vi "measureEchoes_anySet.vi"(3 "Read freqs. \nfrom textfile":bool, 5 "Cluster":T1={"span"=600000000.0, "rbw"=1000.0, "enableVBW"=FALSE, "vbw"=0.0, "traceLength"=64001, "window"=0, "verticalUnit"=0, "center freq"=300000000.0} {"verticalUnit" items=["SpectrumVerticalUnit_dBm", "SpectrumVerticalUnit_Watt", "SpectrumVerticalUnit_Volt", "SpectrumVerticalUnit_Amp", "SpectrumVerticalUnit_dBmV"]; "window" items=["SpectrumWindow_Kaiser", "SpectrumWindow_Mil6dB", "SpectrumWindow_BlackmanHarris", "SpectrumWindow_Rectangle", "SpectrumWindow_FlatTop", "SpectrumWindow_Hann"]; "traceLength" items=["801"=801, "2401"=2401, "4001"=4001, "8001"=8001, "10401"=10401, "16001"=16001, "32001"=32001, "64001"=64001]}, 6 "error in":errorcluster, 7 "Echo measurement time":i32=30, 8 "Burn time/OFC measurement time":i32=30, 9 "Folder for all data (Don't forget the last slash!)":string) -> (0 "error out":errorcluster)   [LabVIEW 2016]
uses:
  <vilib>/Utility/file.llb/Read Delimited Spreadsheet (DBL).vi
  <vilib>/Utility/file.llb/Write Delimited Spreadsheet (DBL).vi
panel:
  out "Last saved trace":sgl[](graph)
  in  "stop":bool
  out "RSA error out":errorcluster
  out "Real-time trace":sgl[](graph)
  out "Current set #":i32
  out "Current freq.":dbl
  in  "freqs. file":path
  in  "Shuffle?":bool
  in  "Start freq":dbl=100000.0 format="%0.2e"
  in  "End freq":dbl=20000000.0 format="%0.2e"
  in  "Freq step":i32=100000 format="%.2e"
  in  "Mod shape":enum16{"Triangle", "Sine"}(ring)
  # "RSA settings"
  # "Suppose you want to collect comb data, first ascending, then descending.\n\nIn Matlab, create a 1xM array \ncontaining all modulation freqs (Hz) in the ascending sequence; then create a 1xN array for the descending case. Note that M != N is fine.\n\nfid= fopen(FILENAME, 'w');\nfprintf(fid,'%d\\t', ARRAY1);\nfprintf(fid,'\\r\\n');\nfprintf(fid,'%d\\t',ARRAY2);\n... \n(for more sets, repeat as needed)\nfclose(fid);\n\nNow find the file you just made:"
  # "Modulation settings"
  # "(zero-indexed)"
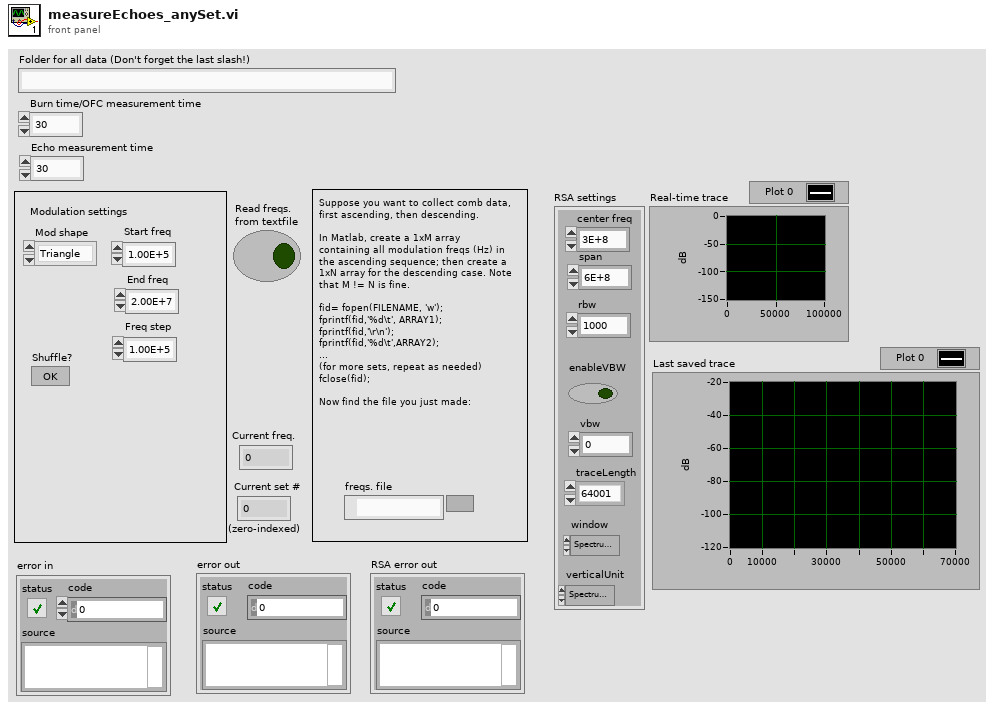
[diagram p1: front panel]
types:
  T1 = cluster{"span":dbl, "rbw":dbl, "enableVBW":bool, "vbw":dbl, "traceLength":u16, "window":u32, "verticalUnit":u32, "center freq":dbl}
  T2 = cluster{"span":dbl, "rbw":dbl, "enableVBW":bool, "vbw":dbl, "traceLength":u16, "window":u32, "verticalUnit":u32}
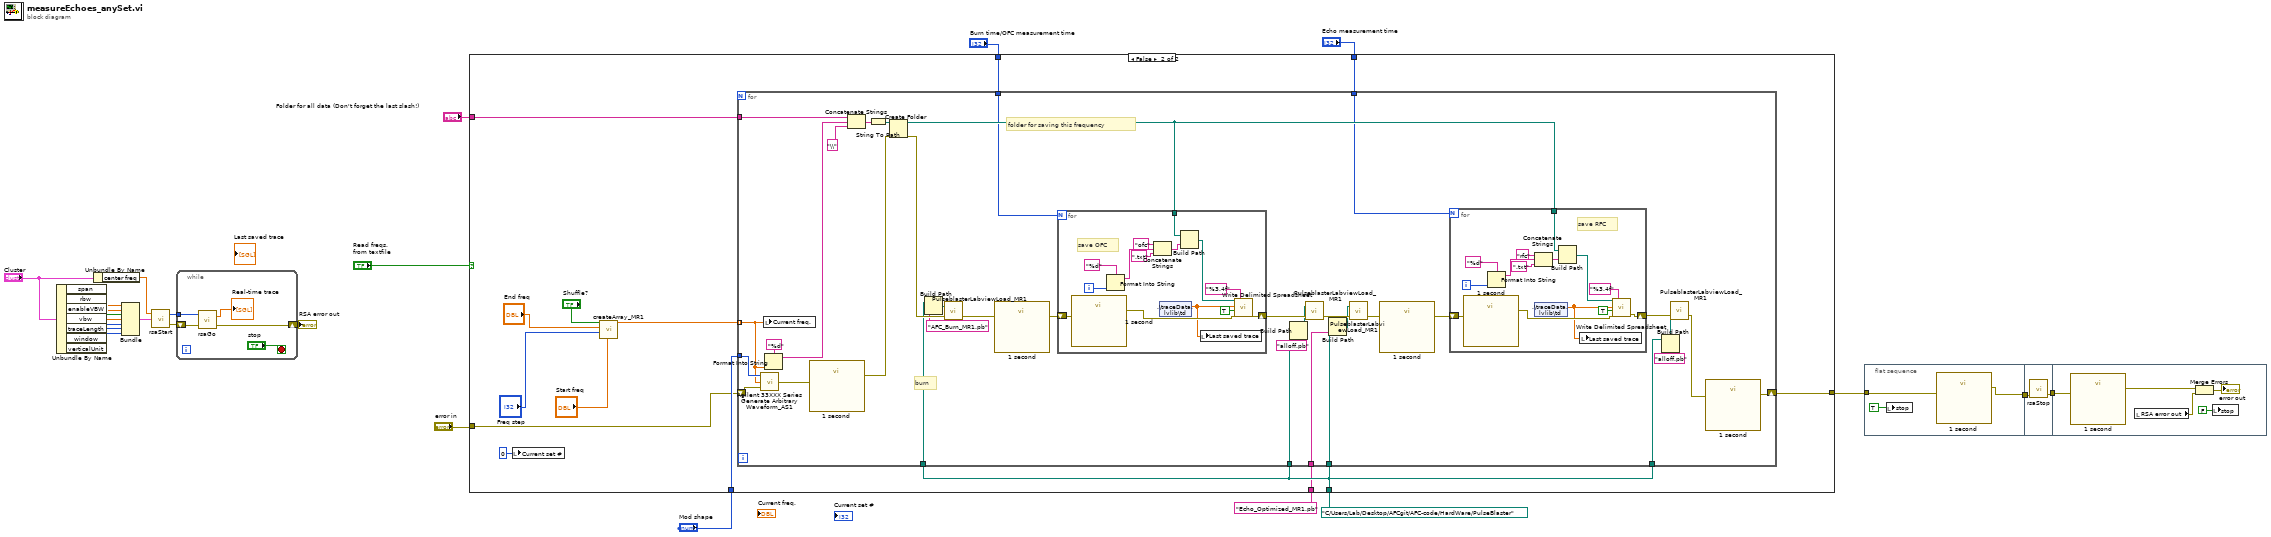
[diagram p0: block diagram]
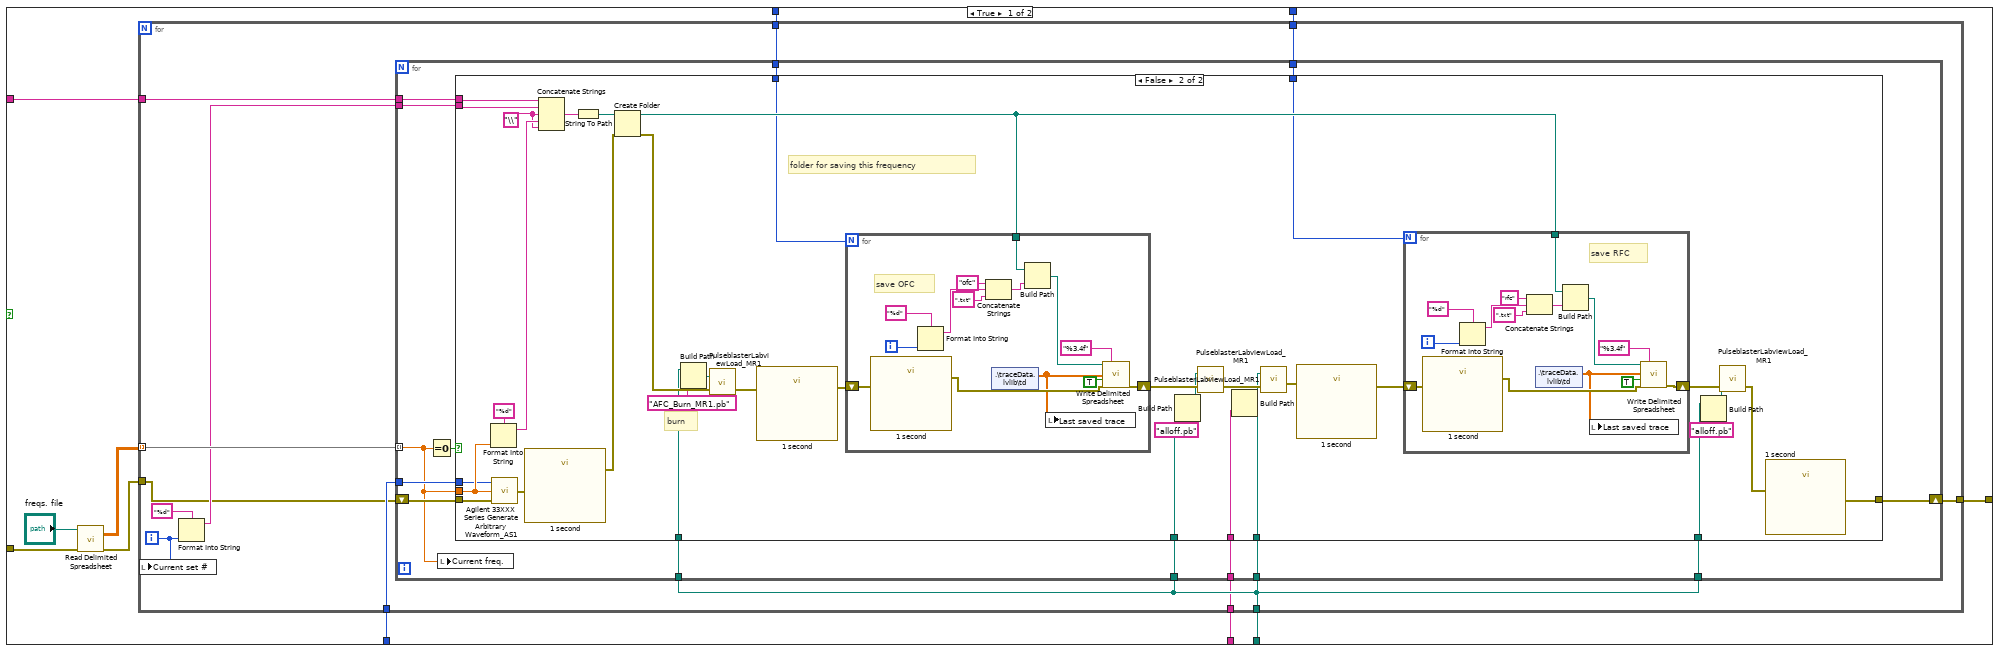
[diagram p2: hidden frame]
diagram:
  n1 = Unbundle By Name("Cluster") -> ("span"=w17:dbl, "rbw"=w18:dbl, "enableVBW"=w19:bool, "vbw"=w20:dbl, "traceLength"=w21:u16, "window"=w22:u32, "verticalUnit"=w23:u32)
  n2 = Unbundle By Name("Cluster") -> ("center freq"=w10:dbl)
  n3 = Bundle("span"=w17, "rbw"=w18, "enableVBW"=w19, "vbw"=w20, "traceLength"=w21, "window"=w22, "verticalUnit"=w23) -> (w9:T2)  [unwired: 1 in]
  n4 = call "rsaStart.vi"("Cluster"=w9, "center freq"=w10) -> ("error out"=w7:errorcluster, "traceLength"=w8:u16)  [unwired: 1 in]
  n5 = while {
    tunnel: w8 -> [w29]
    shift-right: [w27] -> w6
    shift-left: w7 -> [w26]
    stop <- "stop" stop-if-true
    n6 = call "rsaGo.vi"("error in"=w26, "Trace length"=w29) -> ("error out"=w27:errorcluster, "traceData out"=→"Real-time trace":sgl[])  [unwired: 1 in]
  }
  "RSA error out" <- w6
  n7 = case shown="False" "Read freqs. \nfrom textfile" {
    tunnel: "Folder for all data (Don't forget the last slash!)" -> [w40 w146]
    tunnel: path "C:/Users/Lab/Desktop/AFCgit/AFC-code/HardWare/PulseBlaster" ("base path") -> [w32 w145]
    tunnel: "Burn time/OFC measurement time" -> [w39 w144]
    tunnel: "Echo measurement time" -> [w38 w143]
    tunnel: "error in" -> [w36 w134]
    tunnel: "Mod shape" -> [w33 w137]
    tunnel: [w31 w135] -> w24
    tunnel: "Echo_Optimized_MR1.pb" ("name or relative path") -> [w30 w133]
    frame True {
      n8 = call-poly <vilib>:"Read Delimited Spreadsheet.vi"("file path (dialog if empty)"="freqs. file", "error in (no error)"=w36) -> ("all rows"=w35:dbl[][], "error out"=w34:errorcluster)  [unwired: 8 in, 4 out]
      n9 = for {
        tunnel: [w52] -> w31
        tunnel: w40 -> [w51]
        tunnel: w32 -> [w50]
        tunnel: w39 -> [w49]
        tunnel: w38 -> [w48]
        tunnel: w35 -> [w47] mode=indexing
        tunnel: w34 -> [w42]
        tunnel: w33 -> [w44]
        tunnel: w30 -> [w41]
        i -> [w43]
        n10 = local write "Current set #"(w43) -> ()
        n11 = Format Into String(format string="%d", w43) -> (resulting string=w45:string)  [unwired: 2 in, 1 out]
        n12 = for {
          tunnel: w47 -> [w54] mode=indexing
          tunnel: w44 -> [w66]
          shift-right: [w65] -> w52
          shift-left: w42 -> [w64]
          tunnel: w51 -> [w56]
          tunnel: w50 -> [w63]
          tunnel: w50 -> [w62]
          tunnel: w50 -> [w61]
          tunnel: w50 -> [w60]
          tunnel: w49 -> [w59]
          tunnel: w48 -> [w58]
          tunnel: w45 -> [w57]
          tunnel: w41 -> [w53]
          n13 = Equal To 0?(x=w54) -> (x = 0?=w55:bool)
          n14 = local write "Current freq."(w54) -> ()
          n15 = case shown="False" w55 {
            tunnel: w66 -> [_ w75]
            tunnel: [w67 w69] -> w65
            tunnel: w64 -> [w67 w77]
            tunnel: w63 -> [_ w96]
            tunnel: w62 -> [_ w93]
            tunnel: w61 -> [_ w91]
            tunnel: w60 -> [_ w88]
            tunnel: w59 -> [_ w86]
            tunnel: w58 -> [_ w85]
            tunnel: w57 -> [_ w80]
            tunnel: w56 -> [_ w81]
            tunnel: w54 -> [_ w76]
            tunnel: w53 -> [_ w68]
            frame True {
            }
            frame False {
              w83 = "\\" ("string")
              # "folder for saving this frequency"
              # "burn"
              n16 = Format Into String(format string="%d", w76) -> (resulting string=w84:string)  [unwired: 2 in, 1 out]
              n17 = call "Agilent 33XXX Series Generate Arbitrary Waveform_AS1.vi"("error in (no error)"=w77, "Frequency (1000 Hz)"=w76, "Enum"=w75) -> ("error out"=w78:errorcluster)
              n18 = call "1 second"("error in (no error)"=w78) -> ("error out"=w100:errorcluster)  [unwired: 10 in]
              n19 = Concatenate Strings(w81, w80, w83, w84, w83) -> (w79:string)
              n20 = String To Path(string=w79) -> (path=w97:path)
              n21 = Create Folder(path (use dialog)=w97, error in=w100) -> (created path=w98:path, error out=w99:errorcluster)  [unwired: 1 in, 1 out]
              n22 = Build Path(base path=w96, name or relative path="AFC_Burn_MR1.pb") -> (appended path=w94:path)
              n23 = call "PulseblasterLabviewLoad_MR1.vi"("error in (no error)"=w99, "Input file"=w94) -> ("error out"=w74:errorcluster)  [unwired: 1 out]
              n24 = call "1 second"("error in (no error)"=w74) -> ("error out"=w73:errorcluster)  [unwired: 10 in]
              n25 = for {
                N: w86 -> [_]
                shift-right: [w131] -> w101
                shift-left: w73 -> [w121]
                tunnel: w98 -> [w124]
                i -> [w122]
                # "save OFC"
                n26 = call "1 second"("error in (no error)"=w121) -> ("error out"=w120:errorcluster)  [unwired: 10 in]
                n27 = Format Into String(format string="%d", w122) -> (resulting string=w127:string)  [unwired: 2 in, 1 out]
                n28 = Concatenate Strings("ofc" ("string"), w127, ".txt" ("string")) -> (w126:string)
                n29 = shared-variable ".\\traceData.lvlib\\td"() -> (w119:dbl[])  [unwired: 1 in, 1 out]
                n30 = Build Path(base path=w124, name or relative path=w126) -> (appended path=w130:path)
                n31 = local write "Last saved trace"(w119) -> ()
                n32 = call-poly <vilib>:"Write Delimited Spreadsheet.vi"("file path (dialog if empty)"=w130, "format (%.3f)"="%3.4f", "1D data"=w119, "append to file? (new file:F)"=TRUE, "error in (no error)"=w120) -> ("error out"=w131:errorcluster)  [unwired: 9 in, 1 out]
              }
              n33 = Build Path(base path=w91, name or relative path="alloff.pb") -> (appended path=w90:path)
              n34 = call "PulseblasterLabviewLoad_MR1.vi"("error in (no error)"=w101, "Input file"=w90) -> ("error out"=w102:errorcluster)  [unwired: 1 out]
              n35 = Build Path(base path=w93, name or relative path=w68) -> (appended path=w92:path)
              n36 = call "PulseblasterLabviewLoad_MR1.vi"("error in (no error)"=w102, "Input file"=w92) -> ("error out"=w72:errorcluster)  [unwired: 1 out]
              n37 = call "1 second"("error in (no error)"=w72) -> ("error out"=w71:errorcluster)  [unwired: 10 in]
              n38 = for {
                N: w85 -> [_]
                shift-right: [w117] -> w103
                shift-left: w71 -> [w107]
                tunnel: w98 -> [w109]
                i -> [w113]
                # "save RFC"
                n39 = call "1 second"("error in (no error)"=w107) -> ("error out"=w106:errorcluster)  [unwired: 10 in]
                n40 = Format Into String(format string="%d", w113) -> (resulting string=w112:string)  [unwired: 2 in, 1 out]
                n41 = Concatenate Strings("rfc" ("string"), w112, ".txt" ("string")) -> (w111:string)
                n42 = shared-variable ".\\traceData.lvlib\\td"() -> (w105:dbl[])  [unwired: 1 in, 1 out]
                n43 = Build Path(base path=w109, name or relative path=w111) -> (appended path=w116:path)
                n44 = local write "Last saved trace"(w105) -> ()
                n45 = call-poly <vilib>:"Write Delimited Spreadsheet.vi"("file path (dialog if empty)"=w116, "format (%.3f)"="%3.4f", "1D data"=w105, "append to file? (new file:F)"=TRUE, "error in (no error)"=w106) -> ("error out"=w117:errorcluster)  [unwired: 9 in, 1 out]
              }
              n46 = Build Path(base path=w88, name or relative path="alloff.pb") -> (appended path=w87:path)
              n47 = call "PulseblasterLabviewLoad_MR1.vi"("error in (no error)"=w103, "Input file"=w87) -> ("error out"=w70:errorcluster)  [unwired: 1 out]
              n48 = call "1 second"("error in (no error)"=w70) -> ("error out"=w69:errorcluster)  [unwired: 10 in]
            }
          }
        }
      }
    }
    frame False {
      n49 = local write "Current set #"(0 ("Current set #")) -> ()
      n50 = call "createArray_MR1.vi"("Start freq"="Start freq", "Freq step"="Freq step", "End freq"="End freq", "Shuffle?"="Shuffle?") -> ("Riffled {X}"=w138:dbl[])  [unwired: 7 in]
      n51 = for {
        tunnel: w138 -> [w155] mode=indexing
        tunnel: w137 -> [w182]
        shift-right: [w150] -> w135
        shift-left: w134 -> [w181]
        tunnel: w146 -> [w158]
        tunnel: w145 -> [w168]
        tunnel: w145 -> [w165]
        tunnel: w145 -> [w163]
        tunnel: w145 -> [w160]
        tunnel: w144 -> [w157]
        tunnel: w143 -> [w156]
        tunnel: w133 -> [w147]
        # "folder for saving this frequency"
        # "burn"
        n52 = call "Agilent 33XXX Series Generate Arbitrary Waveform_AS1.vi"("error in (no error)"=w181, "Frequency (1000 Hz)"=w155, "Enum"=w182) -> ("error out"=w177:errorcluster)
        n53 = local write "Current freq."(w155) -> ()
        n54 = Format Into String(format string="%d", w155) -> (resulting string=w179:string)  [unwired: 2 in, 1 out]
        n55 = call "1 second"("error in (no error)"=w177) -> ("error out"=w173:errorcluster)  [unwired: 10 in]
        n56 = Concatenate Strings(w158, w179, "\\" ("string")) -> (w170:string)
        n57 = String To Path(string=w170) -> (path=w169:path)
        n58 = Create Folder(path (use dialog)=w169, error in=w173) -> (created path=w171:path, error out=w172:errorcluster)  [unwired: 1 in, 1 out]
        n59 = Build Path(base path=w168, name or relative path="AFC_Burn_MR1.pb") -> (appended path=w166:path)
        n60 = call "PulseblasterLabviewLoad_MR1.vi"("error in (no error)"=w172, "Input file"=w166) -> ("error out"=w152:errorcluster)  [unwired: 1 out]
        n61 = call "1 second"("error in (no error)"=w152) -> ("error out"=w153:errorcluster)  [unwired: 10 in]
        n62 = for {
          N: w157 -> [_]
          shift-right: [w209] -> w174
          shift-left: w153 -> [w199]
          tunnel: w171 -> [w202]
          i -> [w200]
          # "save OFC"
          n63 = call "1 second"("error in (no error)"=w199) -> ("error out"=w198:errorcluster)  [unwired: 10 in]
          n64 = Format Into String(format string="%d", w200) -> (resulting string=w205:string)  [unwired: 2 in, 1 out]
          n65 = Concatenate Strings("ofc" ("string"), w205, ".txt" ("string")) -> (w204:string)
          n66 = shared-variable ".\\traceData.lvlib\\td"() -> (w197:dbl[])  [unwired: 1 in, 1 out]
          n67 = Build Path(base path=w202, name or relative path=w204) -> (appended path=w208:path)
          n68 = local write "Last saved trace"(w197) -> ()
          n69 = call-poly <vilib>:"Write Delimited Spreadsheet.vi"("file path (dialog if empty)"=w208, "format (%.3f)"="%3.4f", "1D data"=w197, "append to file? (new file:F)"=TRUE, "error in (no error)"=w198) -> ("error out"=w209:errorcluster)  [unwired: 9 in, 1 out]
        }
        n70 = Build Path(base path=w163, name or relative path="alloff.pb") -> (appended path=w162:path)
        n71 = call "PulseblasterLabviewLoad_MR1.vi"("error in (no error)"=w174, "Input file"=w162) -> ("error out"=w175:errorcluster)  [unwired: 1 out]
        n72 = Build Path(base path=w165, name or relative path=w147) -> (appended path=w164:path)
        n73 = call "PulseblasterLabviewLoad_MR1.vi"("error in (no error)"=w175, "Input file"=w164) -> ("error out"=w148:errorcluster)  [unwired: 1 out]
        n74 = call "1 second"("error in (no error)"=w148) -> ("error out"=w149:errorcluster)  [unwired: 10 in]
        n75 = for {
          N: w156 -> [_]
          shift-right: [w195] -> w176
          shift-left: w149 -> [w185]
          tunnel: w171 -> [w187]
          i -> [w191]
          # "save RFC"
          n76 = call "1 second"("error in (no error)"=w185) -> ("error out"=w184:errorcluster)  [unwired: 10 in]
          n77 = Format Into String(format string="%d", w191) -> (resulting string=w190:string)  [unwired: 2 in, 1 out]
          n78 = Concatenate Strings("rfc" ("string"), w190, ".txt" ("string")) -> (w189:string)
          n79 = shared-variable ".\\traceData.lvlib\\td"() -> (w183:dbl[])  [unwired: 1 in, 1 out]
          n80 = Build Path(base path=w187, name or relative path=w189) -> (appended path=w194:path)
          n81 = local write "Last saved trace"(w183) -> ()
          n82 = call-poly <vilib>:"Write Delimited Spreadsheet.vi"("file path (dialog if empty)"=w194, "format (%.3f)"="%3.4f", "1D data"=w183, "append to file? (new file:F)"=TRUE, "error in (no error)"=w184) -> ("error out"=w195:errorcluster)  [unwired: 9 in, 1 out]
        }
        n83 = Build Path(base path=w160, name or relative path="alloff.pb") -> (appended path=w159:path)
        n84 = call "PulseblasterLabviewLoad_MR1.vi"("error in (no error)"=w176, "Input file"=w159) -> ("error out"=w151:errorcluster)  [unwired: 1 out]
        n85 = call "1 second"("error in (no error)"=w151) -> ("error out"=w150:errorcluster)  [unwired: 10 in]
      }
    }
  }
  n86 = flat-sequence {
    tunnel: w24 -> [w212]
    tunnel: [w211] -> w5
    tunnel: w5 -> [w215]
    tunnel: [w214] -> w4
    tunnel: w4 -> [w217]
    frame #0 {
      n87 = local write "stop"(TRUE ("Stop")) -> ()
      n88 = call "1 second"("error in (no error)"=w212) -> ("error out"=w211:errorcluster)  [unwired: 10 in]
    }
    frame #1 {
      n89 = call "rsaStop.vi"("error in (no error)"=w215) -> ("error out"=w214:errorcluster)  [unwired: 3 in]
    }
    frame #2 {
      n90 = call "1 second"("error in (no error)"=w217) -> ("error out"=w216:errorcluster)  [unwired: 10 in]
      n91 = local read "RSA error out"() -> (w220:errorcluster)
      n92 = Merge Errors(w216, w220) -> (→"error out":errorcluster)
      n93 = local write "stop"(FALSE ("stop")) -> ()
    }
  }
